vi "test_generic.vi"() -> ()   [LabVIEW 2010, in "GenericDisplay.lvclass"]
uses:
  GenericDisplay.lvclass
  main/labview_source/type_definitions/clusters/controls_refs.ctl
  common/classes/ErrorController/ErrorController/ErrorController.lvclass
  common/classes/Image/Image/Image.lvclass
  common/classes/GenericToplevelComponent/GenericToplevelComponent/trigger_type_enum.ctl
  common/classes/ErrorController/ErrorController/class_data.vi
  common/classes/GenericComponent/GenericComponent/GenericComponent.lvclass
panel:
  out "error handler ready?":bool
  in  "number of images":i32=2
  in  "createButton":bool
  out "event handling loop counter":i32=1
  in  "send image":bool
  in  "stop":bool
  # "Test GenericDisplay"
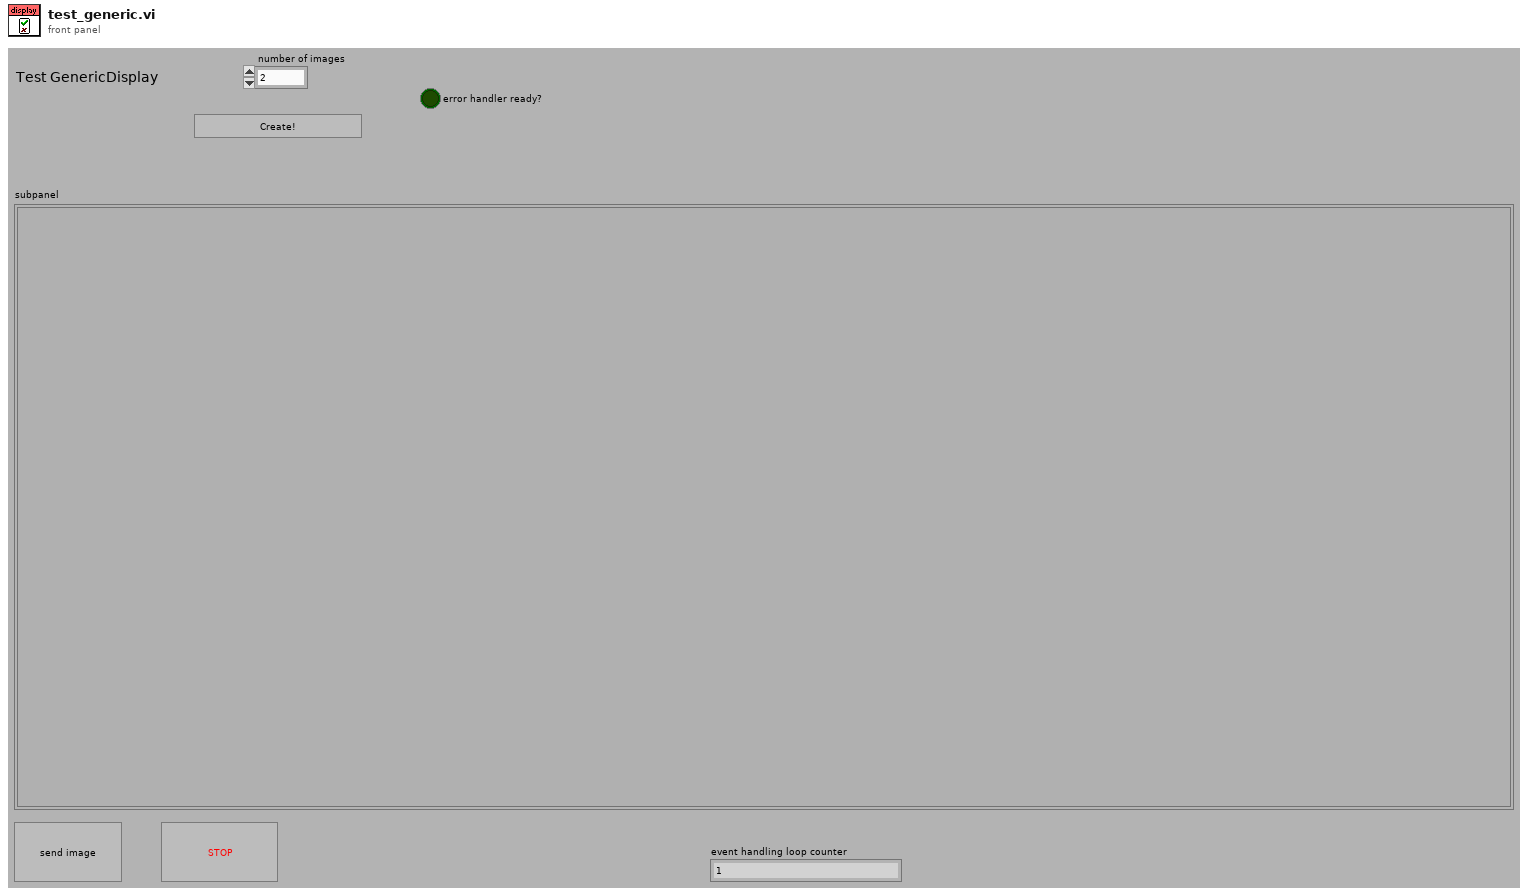
[diagram p1: front panel]
types:
  T1 = typedef "controls_refs.ctl" = cluster{"scan start button":refnum<vi>, "tabs":cluster{"main":refnum<vi>, "settings":refnum<vi>}, "subpanels":cluster{"imagingMode":refnum<vi>, "scanHead":refnum<vi>, "display":refnum<vi>, "experimentController":refnum<vi>, "instrument":refnum<vi>, "stage":refnum<vi>, "stimulator":refnum<vi>, "dataCollection":refnum<vi>, "analyser":refnum<vi>, "daq":refnum<vi>, "imageAssembler":refnum<vi>}, "drop-downs":cluster{"run mode":refnum<vi>, "imagingMode":refnum<vi>, "experimentalController":refnum<vi>, "objective":refnum<vi>}, "status lights":cluster{"experimentController":refnum<vi>, "imagingMode":refnum<vi>, "scanHead":refnum<vi>, "daq":refnum<vi>, "imageAssembler":refnum<vi>, "dataCollection":refnum<vi>, "display":refnum<vi>, "analyser":refnum<vi>, "stage":refnum<vi>, "stimulator":refnum<vi>, "instrument":refnum<vi>}, "message":refnum<vi>, "stimulator enabled?":refnum<vi>, "saving":cluster{"data folder path":refnum<vi>, "file base name":refnum<vi>, "notebook":refnum<vi>}, "progress bar":refnum<vi>, "update icon":refnum<vi>, "title":refnum<vi>, "main vi":refnum<vi>, "user":refnum<vi>, "exit_button":refnum<vi>, "CPU usage %":refnum<vi>}
  T2 = typedef "trigger_type_enum.ctl" = enum8{"external", "internal", "common"}
  T3 = typedef "Image Type" = u32
  T4 = typedef "XComponentSpecification.xctl/data.ctl" = cluster{"class path":string, "configuration":string, "label":string, "settings name":string}
  T5 = typedef "GenericToplevelComponent.lvclass/common_trigger_enum.ctl" = enum16{"NULL", "initialise", "terminate", "fetch command", "fetch data", "attach observer", "register as observer", "detach observer", "acknowledge", "start", "stop", "sweep started", "sweep finished", "experiment started", "experiment stopped"}
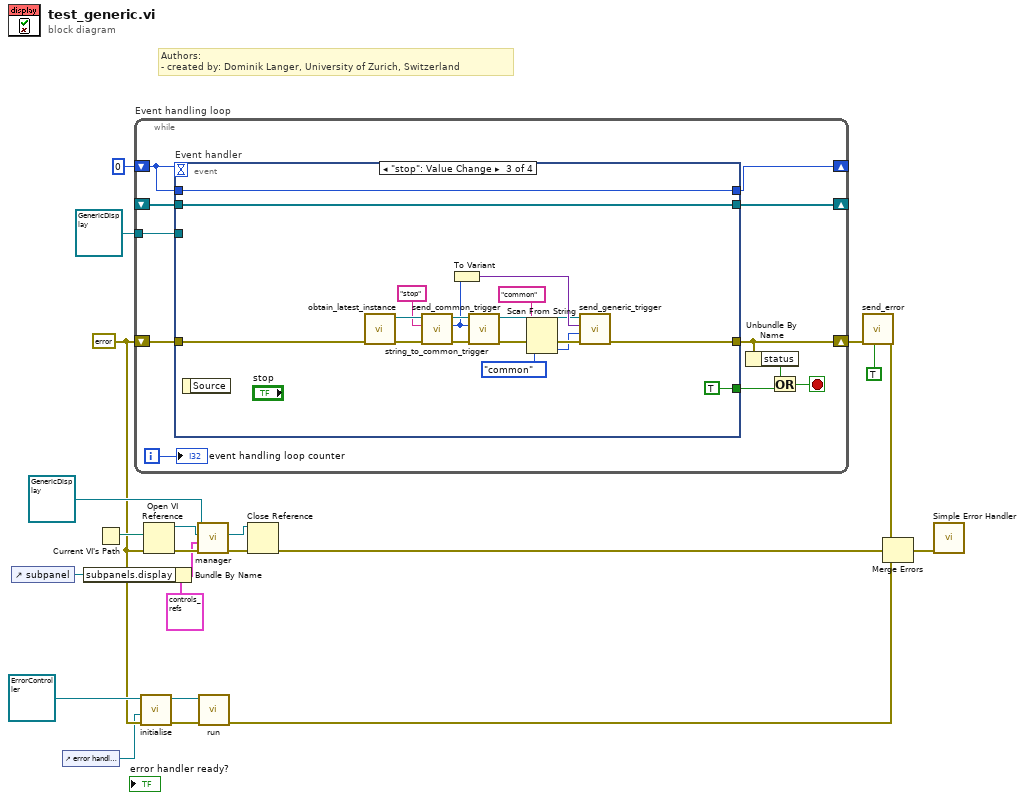
[diagram p0: block diagram]
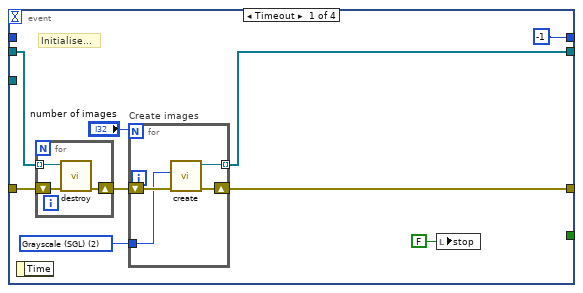
[diagram p2: hidden frame]
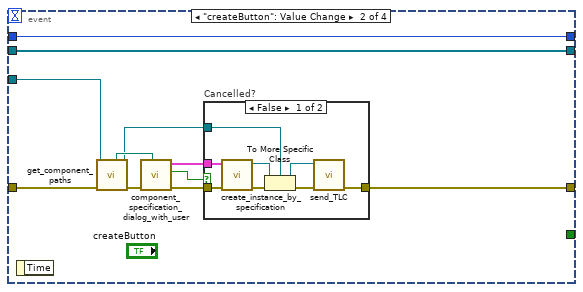
[diagram p3: hidden frame]
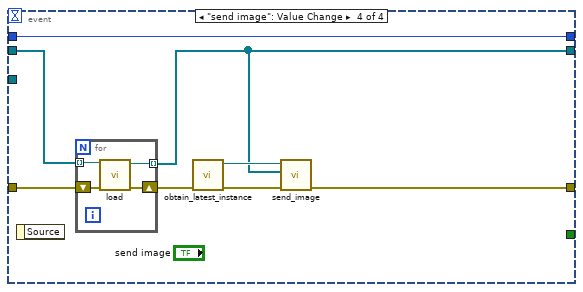
[diagram p5: hidden frame]
diagram:
  w6 = errorcluster {"status"=FALSE, "code"=0, "source"=""} ("error out")
  # "Authors: \n- created by: Dominik Langer, University of Zurich, Switzerland"
  n1 = control-ref of="subpanel"() -> (w21:refnum<vi>)
  n2 = control-ref of="error handler ready?"() -> (w5:refnum<vi>)
  n3 = Bundle By Name(cluster=T1 {"scan start button"=refnum, "tabs"={"main"=refnum, "settings"=refnum}, "subpanels"={"imagingMode"=refnum, "scanHead"=refnum, "display"=refnum, "experimentController"=refnum, "instrument"=refnum, "stage"=refnum, "stimulator"=refnum, "dataCollection"=refnum, "analyser"=refnum, "daq"=refnum, "imageAssembler"=refnum}, "drop-downs"={"run mode"=refnum, "imagingMode"=refnum, "experimentalController"=refnum, "objective"=refnum}, "status lights"={"experimentController"=refnum, "imagingMode"=refnum, "scanHead"=refnum, "daq"=refnum, "imageAssembler"=refnum, "dataCollection"=refnum, "display"=refnum, "analyser"=refnum, "stage"=refnum, "stimulator"=refnum, "instrument"=refnum}, "message"=refnum, "stimulator enabled?"=refnum, "saving"={"data folder path"=refnum, "file base name"=refnum, "notebook"=refnum}, "progress bar"=refnum, "update icon"=refnum, "title"=refnum, "main vi"=refnum, "user"=refnum, "exit_button"=refnum, "CPU usage %"=refnum} ("control references"), "subpanels.display"=w21) -> (w16:T1)
  n4 = Current VI's Path() -> (path=w19:path)
  n5 = while "Event handling loop" {
    shift-right: [w26] -> w10
    shift-left: w6 -> [w33]
    shift-right: [w31] -> _
    shift-left: 0 -> [w32]
    shift-right: [w29] -> _
    shift-left: _ -> [w30]
    tunnel: refnum<class "GenericDisplay.lvclass"> refnum ("GenericDisplay.lvclass") -> [w27]
    i -> [w28]
    stop <- w23 stop-if-true
    n6 = event "Event handler" shown="[2] \"stop\": Value Change" {
      selector: _ -> [_ _ _ _]
      dyn-events: _ -> [_ _ _ _]
      timeout: w32 -> [_ _ _ _]
      tunnel: w33 -> [w40 w54 w84 w93]
      tunnel: [w35 w58 w81 w89] -> w26
      tunnel: [-1 w60 w87 w95] -> w31
      tunnel: w32 -> [_ w60 w87 w95]
      tunnel: [_ _ TRUE _] -> w24
      tunnel: w30 -> [w38 w59 w85 w94]
      tunnel: [w39 w59 w85 w90] -> w29
      tunnel: w27 -> [_ w53 _ _]
      event Timeout {
        w37 = T3 2 items=["Grayscale (U8)", "Grayscale (I16)", "Grayscale (SGL)", "Complex (CSG)", "RGB (U32)", "HSL (U32)", "RGB (U64)", "Grayscale (U16)"] ("Image Type")
        # "Initialise..."
        n7 = event-data() -> ()  [unwired: 2 out]
        n8 = for {
          shift-right: [w48] -> w41
          shift-left: w40 -> [w49]
          tunnel: w38 -> [w47] mode=indexing
          n9 = call-dynamic "destroy.vi"("error in (no error)"=w49, "Image in"=w47) -> ("error out"=w48:errorcluster)  [unwired: 9 out]
        }
        n10 = for "Create images" {
          N: "number of images" -> [_]
          tunnel: [w43] -> w39 mode=indexing
          shift-right: [w45] -> w35
          shift-left: w41 -> [w46]
          tunnel: w37 -> [w44]
          n11 = call "create.vi"("error in (no error)"=w46, "Image Type"=w44) -> ("error out"=w45:errorcluster, "Image out"=w43:refnum<class "Image.lvclass">)  [unwired: 2 in, 6 out]
        }
        n12 = local write "stop"(FALSE ("stop")) -> ()
      }
      event "createButton": Value Change {
        n13 = event-data() -> ()  [unwired: 2 out]
        n14 = call-dynamic "get_component_paths.vi"("error in (no error)"=w54, "GenericComponent in"=w53) -> ("error out"=w57:errorcluster, "GenericComponent out"=w52:refnum<class "GenericDisplay.lvclass">, "component type directory"=w56:path)  [unwired: 4 in, 3 out]
        n15 = call "component_specification_dialog_with_user.vi"("start path"=w56, "error in (no error)"=w57) -> ("error out"=w55:errorcluster, "cancelled?"=w51:bool, "component specification out"=w50:T4)  [unwired: 7 in]
        n16 = case "Cancelled?" shown="False" w51 {
          tunnel: [w65 w69] -> w58
          tunnel: w55 -> [w63 w69]
          tunnel: w52 -> [w62 _]
          tunnel: w50 -> [w61 _]
          frame False {
            n17 = call "create_instance_by_specification.vi"("error in (no error)"=w63, "component specification"=w61) -> ("error out"=w68:errorcluster, "GenericPlugin out"=w67:refnum<class "GenericComponent.lvclass">)  [unwired: 7 in, 1 out]
            n18 = To More Specific Class(target class=w62, reference=w67, error in=w68) -> (specific class reference=w64:refnum<class "GenericDisplay.lvclass">, error out=w66:errorcluster)
            n19 = call-dynamic "send_TLC.vi"("error in (no error)"=w66, "GenericToplevelComponent in"=w64) -> ("error out"=w65:errorcluster)  [unwired: 8 in, 1 out]
          }
          frame True {
          }
        }
      }
      event "stop": Value Change {
        n20 = event-data() -> ()  [unwired: 2 out]
        n21 = call "obtain_latest_instance.vi"("error in (no error)"=w84) -> ("error out"=w78:errorcluster, "GenericDisplay out"=w80:refnum<class "GenericDisplay.lvclass">)  [unwired: 1 in, 8 out]
        n22 = call-dynamic "string_to_common_trigger.vi"("error in (no error)"=w78, "trigger string"="stop", "GenericToplevelComponent in"=w80) -> ("error out"=w77:errorcluster, "trigger"=w70:T5, "GenericToplevelComponent out"=w79:refnum<class "GenericDisplay.lvclass">)  [unwired: 6 in]
        n23 = To Variant(anything=w70) -> (Variant=w83:variant)
        n24 = call-dynamic "send_common_trigger.vi"("error in (no error)"=w77, "trigger"=w70, "GenericToplevelComponent in"=w79) -> ("error out"=w75:errorcluster, "GenericToplevelComponent out"=w82:refnum<class "GenericDisplay.lvclass">)  [unwired: 6 in, 1 out]
        n25 = Scan From String(input string="common", error in=w75, default 1=trigger_type_enum."common" ("trigger type")) -> (error out=w74:errorcluster, output 1=w72:T2)  [unwired: 2 in, 2 out]
        n26 = call-dynamic "send_generic_trigger.vi"("error in (no error)"=w74, "trigger type"=w72, "trigger variant"=w83, "GenericToplevelComponent in"=w82) -> ("error out"=w81:errorcluster)  [unwired: 4 in, 3 out]
      }
      event "send image": Value Change {
        n27 = event-data() -> ()  [unwired: 2 out]
        n28 = for {
          tunnel: w94 -> [w98] mode=indexing
          tunnel: [w97] -> w90 mode=indexing
          shift-right: [w96] -> w92
          shift-left: w93 -> [w99]
          n29 = call-dynamic "load.vi"("error in (no error)"=w99, "Image in"=w98) -> ("error out"=w96:errorcluster, "Image out"=w97:refnum<class "Image.lvclass">)  [unwired: 2 in, 6 out]
        }
        n30 = call "obtain_latest_instance.vi"("error in (no error)"=w92) -> ("error out"=w88:errorcluster, "GenericDisplay out"=w91:refnum<class "GenericDisplay.lvclass">)  [unwired: 1 in, 8 out]
        n31 = call-dynamic "send_image.vi"("error in (no error)"=w88, "image (channels)"=w90, "GenericToplevelComponent in"=w91) -> ("error out"=w89:errorcluster)  [unwired: 6 in, 2 out]
      }
    }
    n32 = Unbundle By Name(w26) -> ("status"=w25:bool)
    n33 = Or(x=w25, y=w24) -> (x .or. y?=w23:bool)
    "event handling loop counter" <- w28
  }
  n34 = call-dynamic "initialise.vi"("error in (no error)"=w6, "error boolean"=w5, "ErrorController in"=refnum<class "ErrorController.lvclass"> refnum ("ErrorController.lvclass")) -> ("error out"=w8:errorcluster, "ErrorController out"=w9:refnum<class "ErrorController.lvclass">)  [unwired: 7 in]
  n35 = Open VI Reference(vi path=w19, error in (no error)=w6) -> (vi reference=w15:refnum<vi>, error out=w17:errorcluster)  [unwired: 4 in]
  n36 = call-dynamic "manager.vi"("error in (no error)"=w17, "control references"=w16, "top-level VI ref in"=w15, "GenericToplevelComponent in"=refnum<class "GenericDisplay.lvclass"> refnum ("GenericDisplay.lvclass")) -> ("error out"=w14:errorcluster, "top-level VI ref out"=w13:refnum<vi>)  [unwired: 5 in, 1 out]
  n37 = call "run.vi"("error in (no error)"=w8, "ErrorController in"=w9) -> ("error out"=w2:errorcluster)  [unwired: 8 in, 1 out]
  n38 = Close Reference(reference=w13, error in (no error)=w14) -> (error out=w3:errorcluster)
  n39 = call "send_error.vi"("last error? (F)"=TRUE, "error in (no error)"=w10) -> ("error out"=w4:errorcluster)  [unwired: 9 in]
  n40 = Merge Errors(w4, w3, w2) -> (w1:errorcluster)
  n41 = call <vilib>:"Simple Error Handler.vi"("error in (no error)"=w1) -> ()  [unwired: 4 in, 5 out]
